vi "ExperimentProgramUI.vi"() -> ()   [LabVIEW 2011]
uses:
  Motors/MotorAxisEnum.ctl
  Motors/MotorPosType.ctl
  Typedefs/XYf.ctl
  Motors/MotorPosFlagsType.ctl
  Typedefs/MeasureConfigOutputMode.ctl
  Typedefs/CmdEnum_UserInterfaceCmd.ctl
  GlobalVariables.vi
panel:
  in  "Run sections util":bool
  in  "Run experiment":bool
  in  "Which motors should the script control?":T1={"Magnet Z"=TRUE, "Magnet rotation"=TRUE, "Camera"={"X"=FALSE, "Y"=FALSE}, "Piezo XY"={"X"=FALSE, "Y"=FALSE}, "Piezo Z"=FALSE}
  in  "Program.Motor Axis accuracy conditions":T2
  out "Simulated positions":T2[](array[typedef])
  in  "Axis to show in graph":T4[](array[typedef])=[enum."magrot", enum."magrot", enum."magpos"]
  out "Positions according to program":dbl[][](graph)
  in  "Tab Control 2":enum32{"Script", "MetaData", "Paths & Settings"}(tab)
  in  "Test run without experiment":bool
  in  "Script":string="% Initial position\n%move magpos 20; move magrot 0;\n%wait\n\n% Program\n%move magrot 1000 speed 100; wait;\n%move magrot 50 speed 10;\n%move magpos 10 speed 2;wait\n"
  in  "Simulate script":bool
  in  "Save script":bool
  in  "Load script":bool
  in  "Description":string
  in  "Project Name":string
  in  "Date":string
  in  "Researcher Name":string
  in  "Bead type":string
  in  "Protocol used":string
  in  "Notes":string
  in  "Write interval [frames]":i32
  in  "Experiment base path":path
  in  "Experiment name":string
  out "Traces will end up here:":path
  in  "Output mode":T5=enum."Track"
  in  "Image output path":string
  in  "Trace output path":string
  in  "Max frames in memory":i32
  out "Approx size in RAM memory:":string
  in  "stop":bool
  # "Axis names:\nmagrot:   Magnet rotation\nmagpos:   Magnet Z (vertical) position\npx, py, pz:   Piezo stage\ncamx, camy: Camera motorized stage\n\nScript events:\nSee bin/Modules/ScriptEventExample.vi"
  # "Instructions:\nmove <axis> <position>;\nMove axis to position at current speed\nmove <axis> <position> speed <speed>;\nMove axis to position at specified speed (units/s)\nidle <seconds>;\nDo nothing for specified time\nsection <optional name>;\nStore current framenumber in section file\nstop;\nStop experiment\nevent <text / parameters>;\nGenerate a script event (see left)"
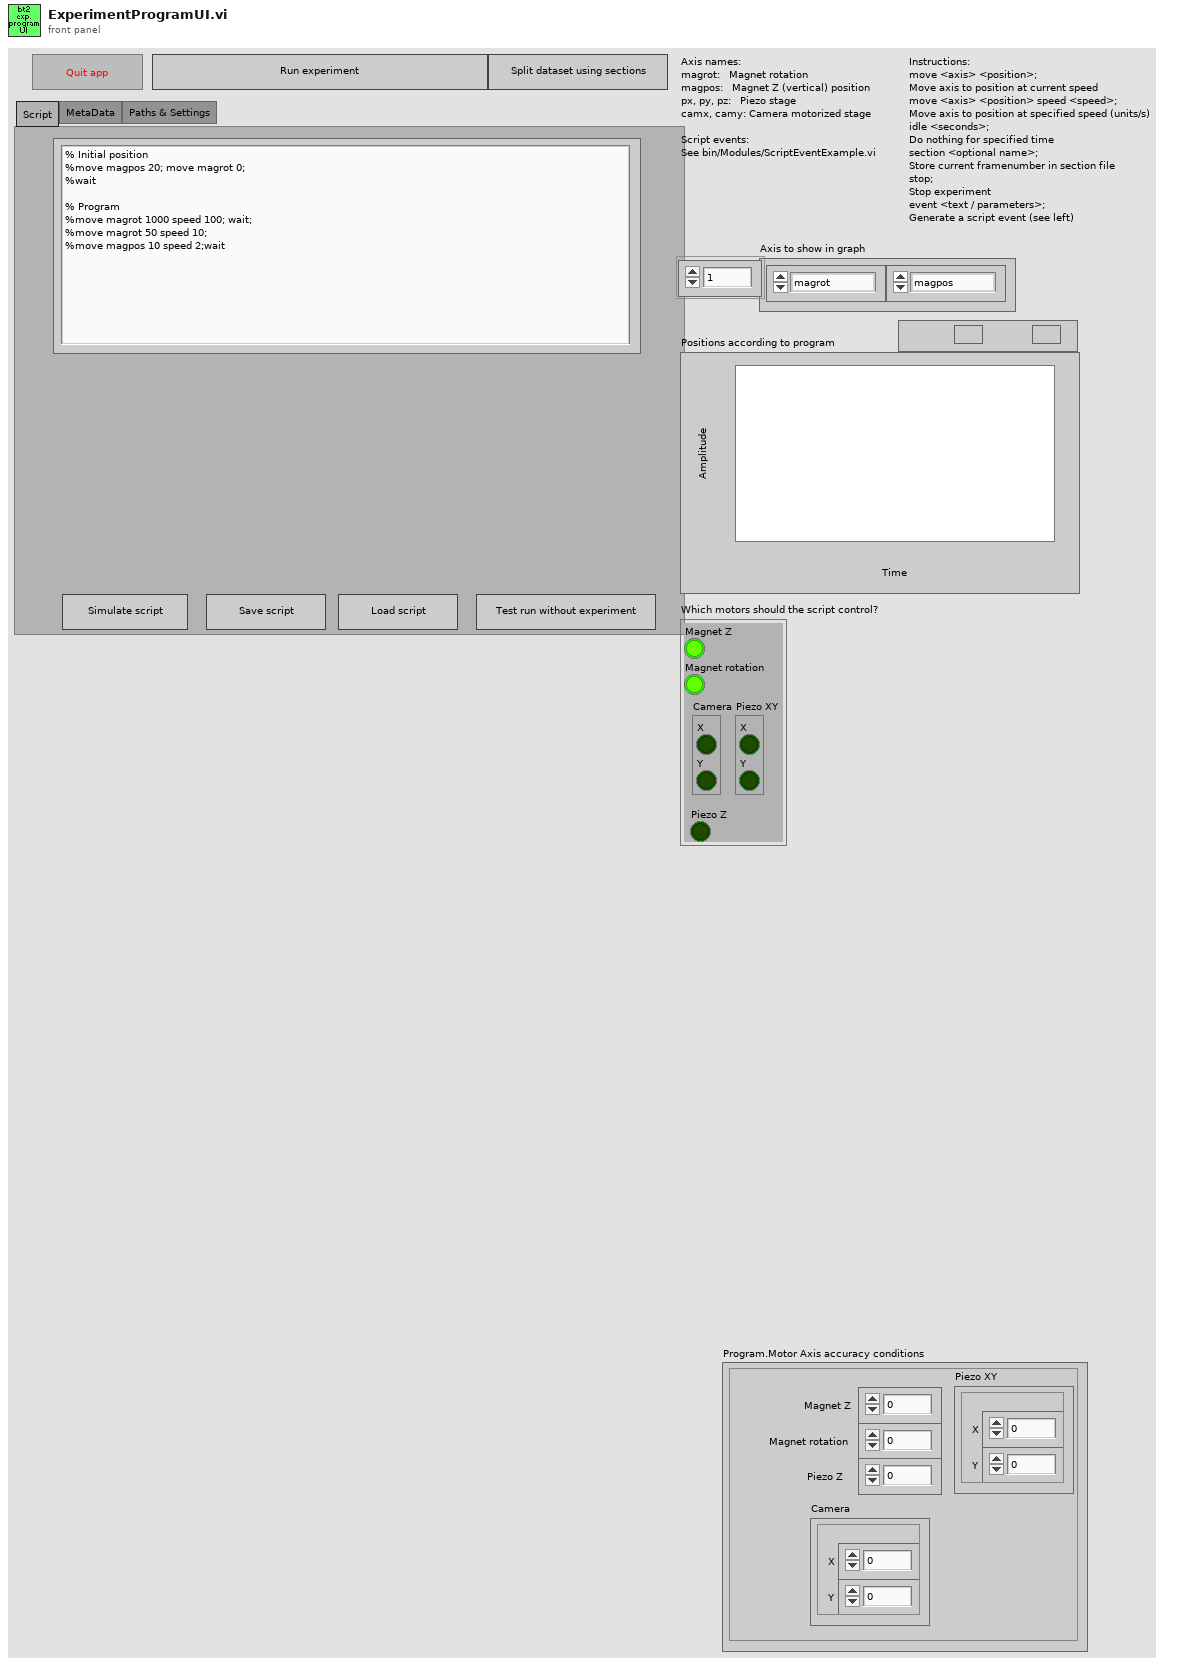
[diagram p1: front panel]
types:
  T1 = typedef "MotorPosFlagsType.ctl" = cluster{"Magnet Z":bool, "Magnet rotation":bool, "Camera":cluster{"X":bool, "Y":bool}, "Piezo XY":cluster{"X":bool, "Y":bool}, "Piezo Z":bool}
  T2 = typedef "MotorPosType.ctl" = cluster{"Magnet Z":dbl, "Magnet rotation":dbl, "Camera":T3, "Piezo XY":T3, "Piezo Z":dbl}
  T3 = typedef "XYf.ctl" = cluster{"X":sgl, "Y":sgl}
  T4 = typedef "MotorAxisEnum.ctl" = enum16{"no axis", "magrot", "magpos", "px", "py", "pz", "camx", "camy"}
  T5 = typedef "MeasureConfigOutputMode.ctl" = enum16{"None", "Track", "SaveImages"}
  T6 = cluster{"UpdateGraphEvent":refnum<user-event>, "MeasureConfigUpdated":refnum<user-event>}
  T7 = typedef "QueueListType.ctl" = cluster{"Motor In":refnum<queue>, "User Interface Image View":refnum<queue>, "User Interface Camera Control":refnum<queue>, "User Interface Event Notifier":refnum<notifier>, "Initialized?":bool, "Experiment Script Event Notifier":refnum<notifier>}
  T8 = typedef "CmdEnum_UserInterfaceCmd.ctl" = enum32{"Idle (Use for default)", "ResultTracesUpdated", "MeasureConfigUpdated", "MeasureEnd", "MeasureStart"}
  T9 = typedef "MeasureConfigType.ctl" = cluster{"Bead locations":cluster{"X":i32, "Y":i32}[], "ROI":i32, "Experiment base path":path, "Image output subdir":string, "Output mode":T5, "Traces output subdir":string, "QTrk Settings":T10, "Tracking Config":T11, "Experiment Name":string, "Program":T14, "ZLUT":sgl[][][], "Camera settings":T17, "Experiment Script":string, "Max frames in memory":i32, "Save traces as binary":bool, "Pixel Calibration Gain Image":string, "Pixel Calibration Offset Image":string, "Use pixel calibration images":bool, "Internal camera settings":string, "Trace write interval":i32, "ExperimentComment":string}
  T10 = typedef "QTrkSettings.ctl" = cluster{"Image width":i32, "Image height":i32, "Number of threads (CPU based)":i32, "CUDA Device":i32, "COM Background correction factor":sgl, "ZLUT MinRadius":sgl, "ZLUT Radial sample density":sgl, "ZLUT Angular sample density":sgl, "ZLUT ROI Coverage":sgl, "QI Iterations":i32, "QI MinRadius":sgl, "QI Radial sample density":sgl, "QI Angular sample density":sgl, "QI ROI Coverage":sgl, "QI Angular Step \nIteration Factor":sgl, "XCOR Profile Length":i32, "XCOR Profile Width":i32, "XCOR Iterations":i32, "Gaussian 2D Fit Iterations":i32, "Gaussian 2D Sigma (pixels)":sgl, "Downsample":i32}
  T11 = typedef "TrackingConfigType.ctl" = cluster{"Number of steps":i32, "ZLUT stepsize (um)":sgl, "Z correction factor":sgl, "Start piezo Z (um)":sgl, "Pixel size (nm)":sgl, "2D Localization Type":T12, "Z Command (None)":T13, "Z Piezo scale":bool, "ZLUT Building\nimages per frame":i32, "ZLUT Bias correction planes":i32}
  T12 = typedef "QTrkLocalizationType.ctl" = enum16{"Center-of-Mass", "1D Cross-Correlation", "Quadrant Interpolation", "Gaussian 2D MLE", "QI + ZLUTAlign", "ZLUTAlign", "QI + FourierLUT"}
  T13 = typedef "QTrkZCommandType.ctl" = enum16{"Nothing", "ComputeZ", "BuildRadialZLUT", "BuildImageZLUT", "RadialZLUT+ImageZLUT"}
  T14 = typedef "ExperimentProgramType.ctl" = cluster{"Commands":T15[], "Motor Axis accuracy conditions":T2, "Axis flags":T1}
  T15 = typedef "ExProgCommandType.ctl" = cluster{"cmd":T16, "axis":T4, "value/pos":dbl, "speed":dbl, "name":string}
  T16 = typedef "ExProgCommandEnumType.ctl" = enum16{"wait", "move", "event", "idle", "when", "section", "stop"}
  T17 = typedef "GenericCameraConfigType.ctl" = cluster{"Framerate (Hz)":i32, "Exposure time (us)":i32, "Image size":cluster{"Width":i32, "Height":i32}, "Number of buffers":i32}
  T18 = typedef "UserInterfaceEventType.ctl" = cluster{"Type":T8}
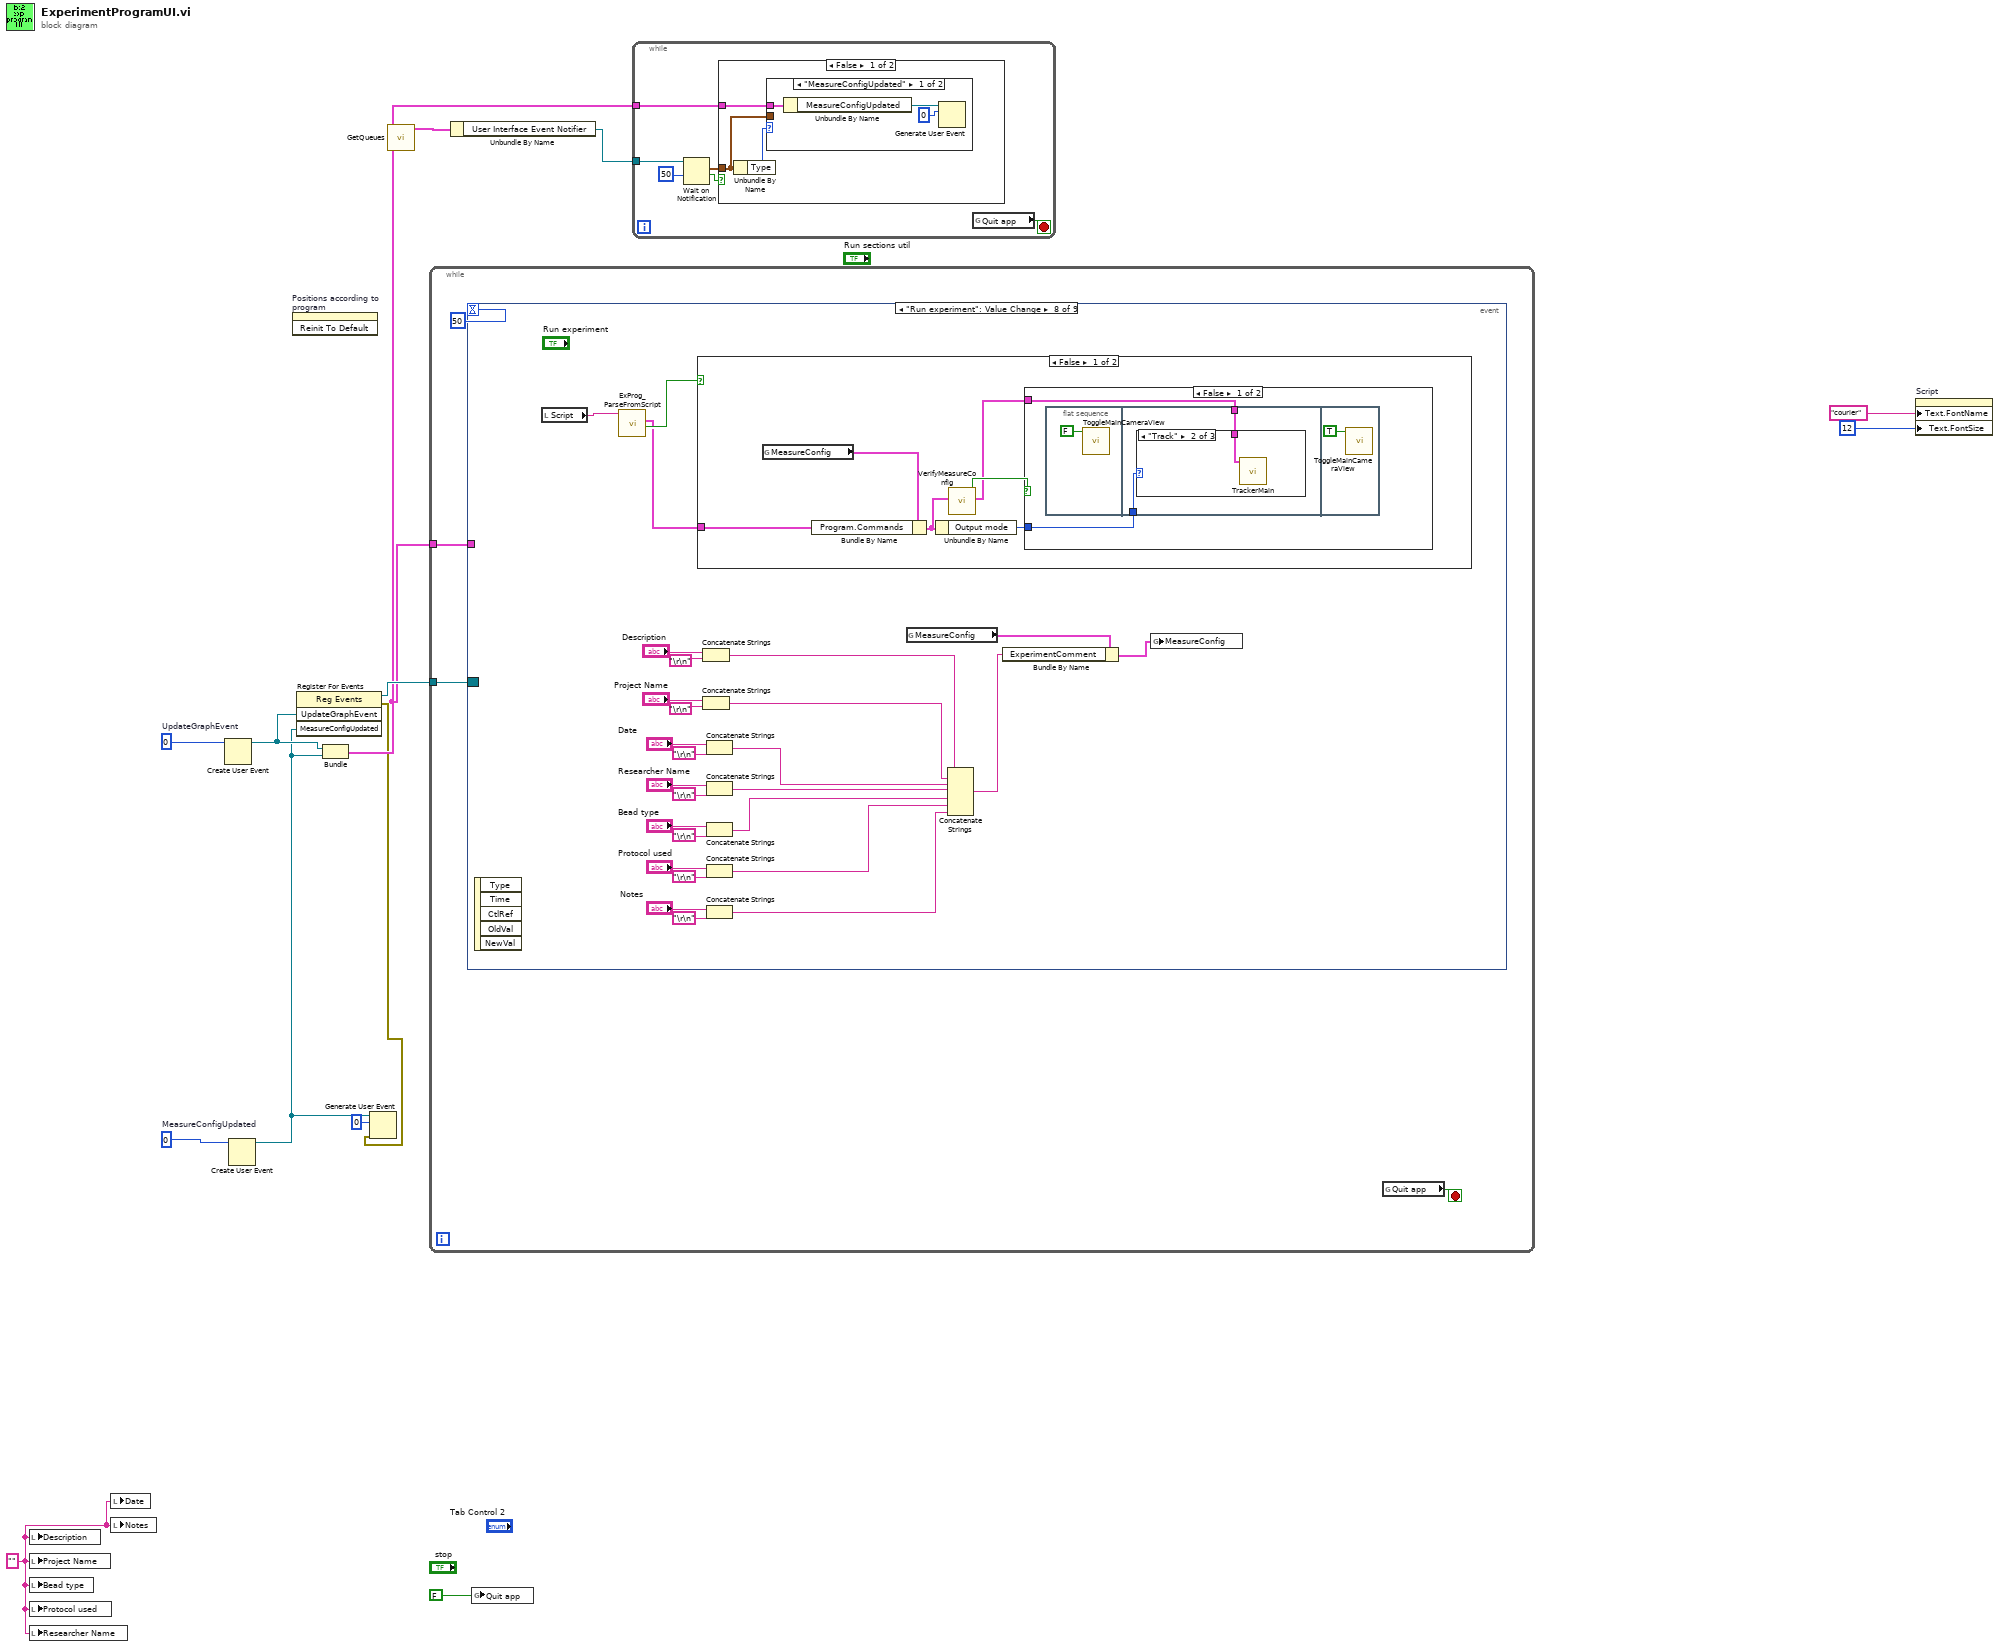
[diagram p0: block diagram]
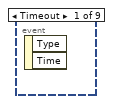
[diagram p4: hidden frame]
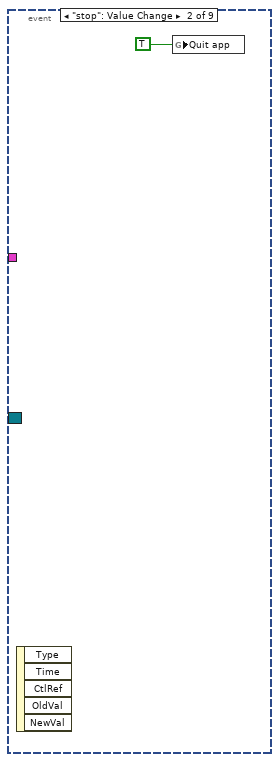
[diagram p5: hidden frame]
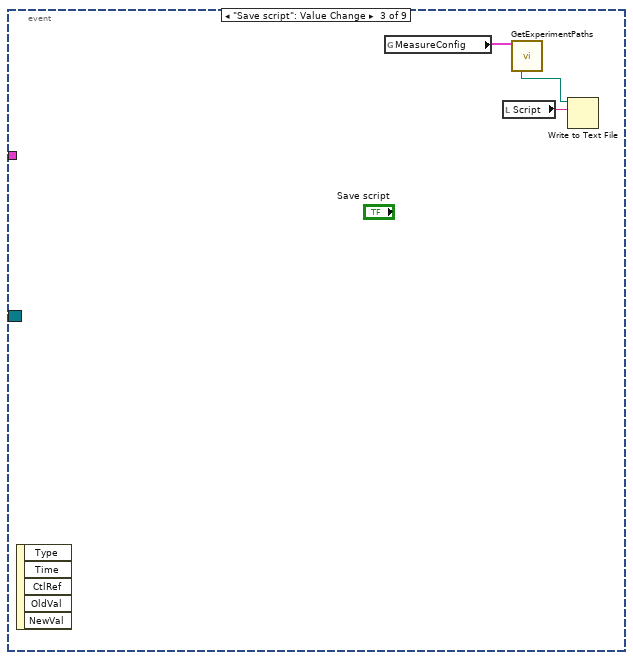
[diagram p6: hidden frame]
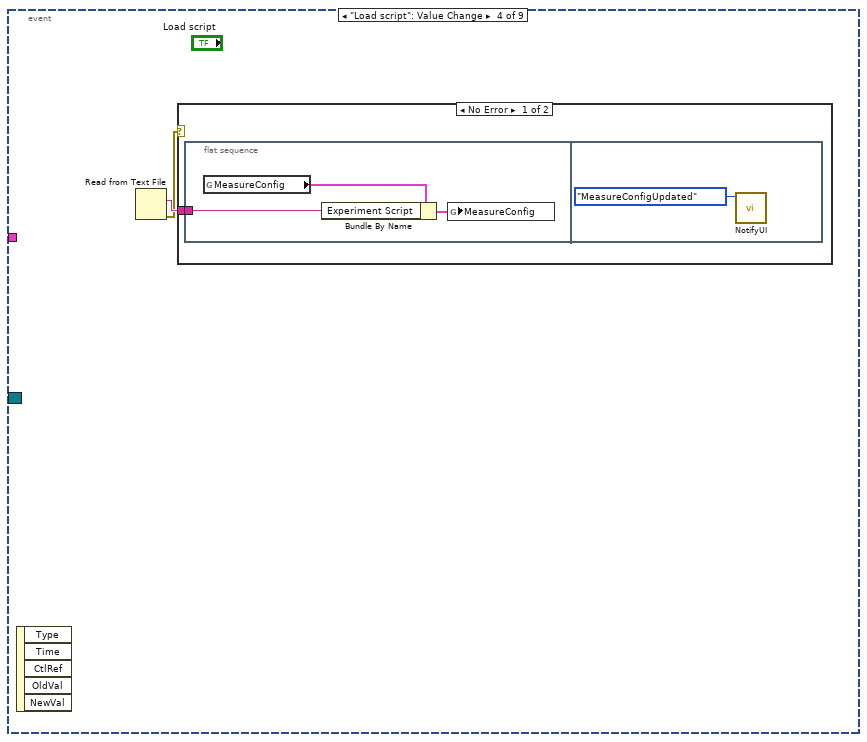
[diagram p7: hidden frame]
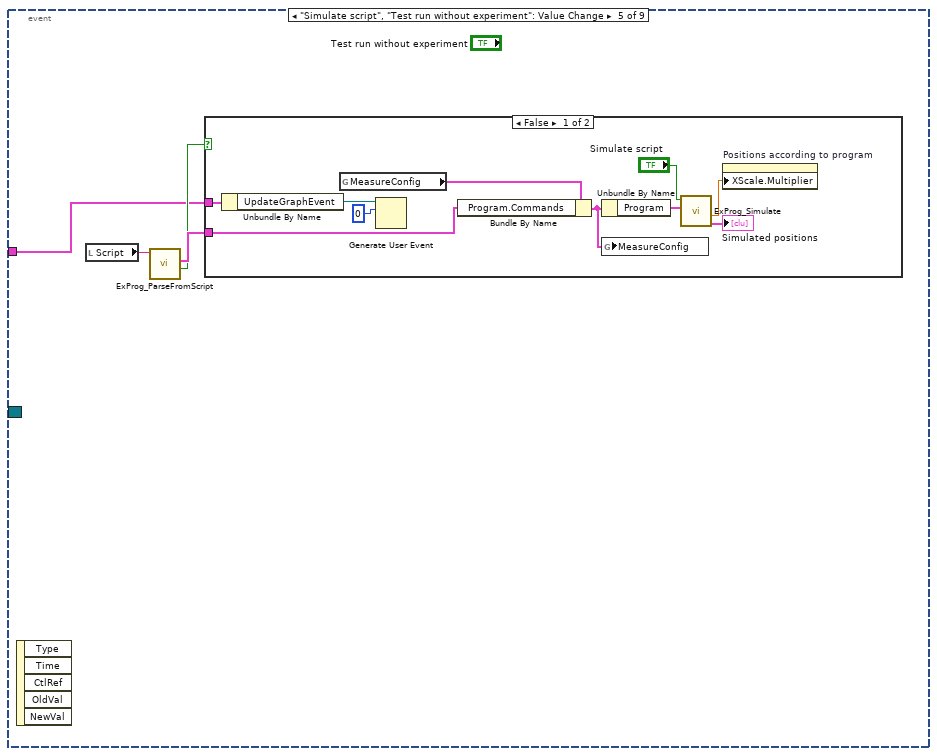
[diagram p9: hidden frame]
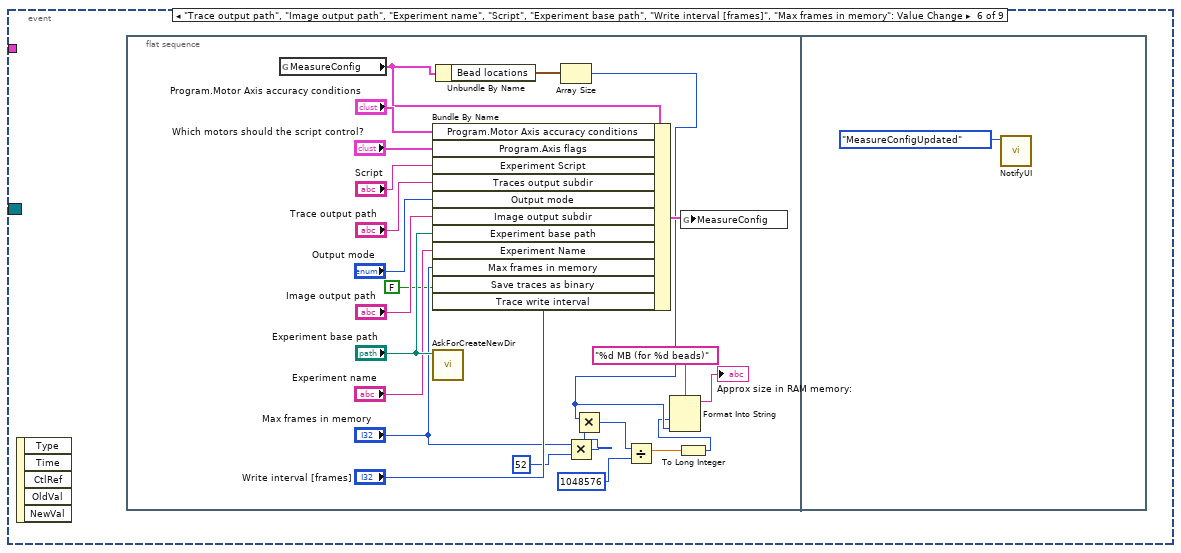
[diagram p11: hidden frame]
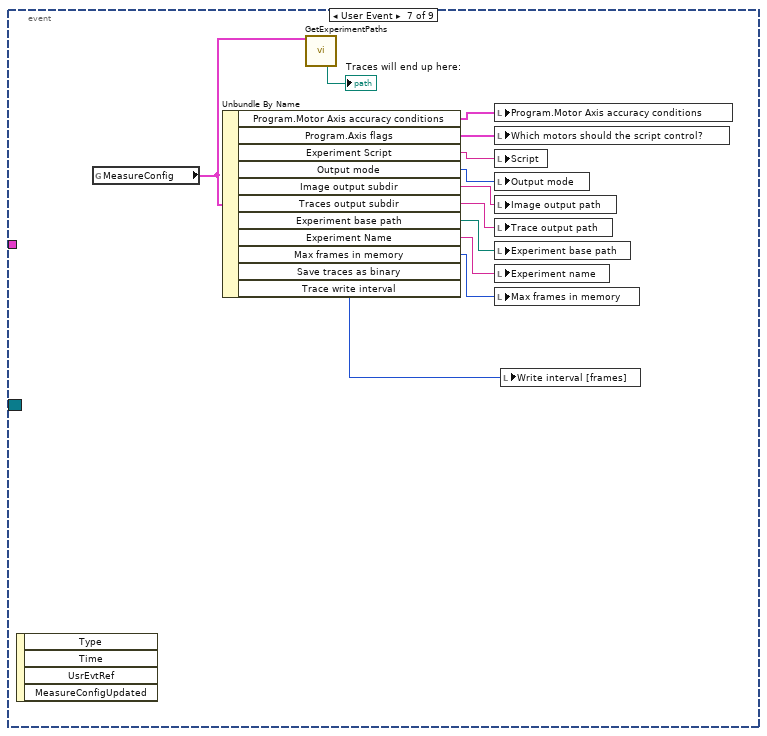
[diagram p12: hidden frame]
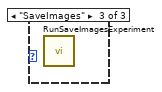
[diagram p14: hidden frame]
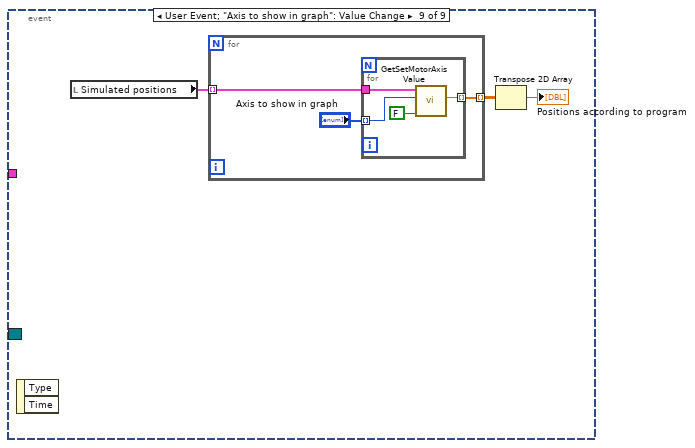
[diagram p17: hidden frame]
diagram:
  w1 = "" ("Description")
  w7 = 0  # MeasureConfigUpdated
  w9 = 0  # UpdateGraphEvent
  n1 = local write "Description"(w1) -> ()
  n2 = local write "Project Name"(w1) -> ()
  n3 = local write "Bead type"(w1) -> ()
  n4 = local write "Protocol used"(w1) -> ()
  n5 = local write "Researcher Name"(w1) -> ()
  n6 = local write "Date"(w1) -> ()
  n7 = local write "Notes"(w1) -> ()
  n8 = Create User Event(user event datatype=w9) -> (user event=w8:refnum<user-event>)  [unwired: 1 in, 1 out]
  n9 = Create User Event(user event datatype=w7) -> (user event=w5:refnum<user-event>)  [unwired: 1 in, 1 out]
  n10 = invoke on="Positions according to program" class="WFGraph (strict)" method="Reinit To Default"() -> ()  [unwired: 3 in, 3 out]
  n11 = register-events(w8, w5) -> (reference out=w10:refnum<event-registration>, error out=w3:errorcluster)  [unwired: 2 in]
  n12 = Bundle("UpdateGraphEvent"=w8, "MeasureConfigUpdated"=w5) -> (w6:T6)  [unwired: 1 in]
  n13 = Generate User Event(user event=w5, event data cluster=0 ("event data"), error in=w3) -> ()  [unwired: 2 out]
  n14 = call "GetQueues.vi"() -> ("Queue List"=w11:T7)  [unwired: 10 in, 1 out]
  n15 = while {
    tunnel: w10 -> [w16]
    tunnel: w6 -> [w15]
    stop <- w18 stop-if-true
    n16 = event shown="[7] \"Run experiment\": Value Change" {
      selector: w16 -> [_ _ _ _ _ _ _ _ _]
      dyn-events: _ -> [_ _ _ _ _ _ _ _ _]
      timeout: 50 -> [_ _ _ _ _ _ _ _ _]
      tunnel: w15 -> [_ _ _ _ w31 _ _ _ _]
      event Timeout {
        n17 = event-data() -> ()  [unwired: 1 in, 2 out]
      }
      event "stop": Value Change {
        n18 = event-data() -> ()  [unwired: 1 in, 5 out]
        n19 = global write "GlobalVariables.vi" "Quit app"(TRUE ("Quit app")) -> ()
      }
      event "Save script": Value Change {
        n20 = event-data() -> ()  [unwired: 1 in, 5 out]
        n21 = global read "GlobalVariables.vi" "MeasureConfig"() -> (w22:T9)
        n22 = local read "Script"() -> (w21:string)
        n23 = call "GetExperimentPaths.vi"("MeasureConfig"=w22) -> ("[base]\\[expname]_script.txt"=w20:path)  [unwired: 6 in, 8 out]
        n24 = Write to Text File(file (use dialog)=w20, text=w21) -> ()  [unwired: 2 in, 3 out]
      }
      event "Load script": Value Change {
        n25 = event-data() -> ()  [unwired: 1 in, 5 out]
        n26 = Read from Text File() -> (text=w24:string, error out=w23:errorcluster)  [unwired: 4 in, 2 out]
        n27 = case shown="No Error" w23 {
          tunnel: w24 -> [w25 _]
          frame No Error {
            n28 = flat-sequence {
              tunnel: w25 -> [w26]
              frame #0 {
                n29 = global read "GlobalVariables.vi" "MeasureConfig"() -> (w27:T9)
                n30 = Bundle By Name(cluster=w27, "Experiment Script"=w26) -> (w28:T9)
                n31 = global write "GlobalVariables.vi" "MeasureConfig"(w28) -> ()
              }
              frame #1 {
                n32 = call "NotifyUI.vi"("User Interface Commands"=CmdEnum_UserInterfaceCmd."MeasureConfigUpdated") -> ()  [unwired: 11 in]
              }
            }
          }
          frame Error {
          }
        }
      }
      event "Simulate script", "Test run without experiment": Value Change {
        n33 = event-data() -> ()  [unwired: 1 in, 5 out]
        n34 = local read "Script"() -> (w30:string)
        n35 = call "ExProg_ParseFromScript.vi"("text"=w30) -> ("error?"=w32:bool, "program"=w33:T15[])  [unwired: 9 in]
        n36 = case shown="False" w32 {
          tunnel: w33 -> [w42 _]
          tunnel: w31 -> [w38 _]
          frame False {
            n37 = Unbundle By Name(w38) -> ("UpdateGraphEvent"=w37:refnum<user-event>)
            n38 = global read "GlobalVariables.vi" "MeasureConfig"() -> (w43:T9)
            n39 = Generate User Event(user event=w37, event data cluster=0 ("event data")) -> ()  [unwired: 1 in, 2 out]
            n40 = Bundle By Name(cluster=w43, "Program.Commands"=w42) -> (w41:T9)
            n41 = Unbundle By Name(w41) -> ("Program"=w40:T14)
            n42 = global write "GlobalVariables.vi" "MeasureConfig"(w41) -> ()
            n43 = call "ExProg_Simulate.vi"("Program"=w40, "Simulation?"="Simulate script") -> ("Wanted position list"=→"Simulated positions":T2[], "Used timestep (s)"=w39:sgl)  [unwired: 8 in]
            n44 = property on="Positions according to program" class="WFGraph (strict)"("XScale.Multiplier"=w39) -> ()  [unwired: 2 in, 2 out]
          }
          frame True {
          }
        }
      }
      event "Trace output path", "Image output path", "Experiment name", "Script", "Experiment base path", "Write interval [frames]", "Max frames in memory": Value Change {
        n45 = event-data() -> ()  [unwired: 1 in, 5 out]
        n46 = flat-sequence {
          frame #0 {
            n47 = global read "GlobalVariables.vi" "MeasureConfig"() -> (w52:T9)
            n48 = Bundle By Name(cluster=w52, "Program.Motor Axis accuracy conditions"="Program.Motor Axis accuracy conditions", "Program.Axis flags"="Which motors should the script control?", "Experiment Script"="Script", "Traces output subdir"="Trace output path", "Output mode"="Output mode", "Image output subdir"="Image output path", "Experiment base path"="Experiment base path", "Experiment Name"="Experiment name", "Max frames in memory"="Max frames in memory", "Save traces as binary"=FALSE, "Trace write interval"="Write interval [frames]") -> (w66:T9)
            n49 = call "AskForCreateNewDir.vi"("Experiment base path"="Experiment base path") -> ()  [unwired: 11 in]
            n50 = Unbundle By Name(w52) -> ("Bead locations"=w51:cluster{"X":i32, "Y":i32}[])
            n51 = Array Size(array=w51) -> (size(s)=w47:i32)
            n52 = Multiply(x="Max frames in memory", y=52) -> (x*y=w50:i32)
            n53 = Multiply(x=w47, y=w50) -> (x*y=w49:i32)
            n54 = Divide(x=w49, y=1048576) -> (x/y=w54:dbl)
            n55 = To Long Integer(number=w54) -> (32bit integer=w46:i32)
            n56 = Format Into String(format string="%d MB (for %d beads)", w46, w47) -> (resulting string=→"Approx size in RAM memory:":string)  [unwired: 2 in, 1 out]
            n57 = global write "GlobalVariables.vi" "MeasureConfig"(w66) -> ()
          }
          frame #1 {
            n58 = call "NotifyUI.vi"("User Interface Commands"=CmdEnum_UserInterfaceCmd."MeasureConfigUpdated") -> ()  [unwired: 11 in]
          }
        }
      }
      event User Event {
        n59 = event-data() -> ()  [unwired: 1 in, 4 out]
        n60 = global read "GlobalVariables.vi" "MeasureConfig"() -> (w73:T9)
        n61 = Unbundle By Name(w73) -> ("Program.Motor Axis accuracy conditions"=w79:T2, "Program.Axis flags"=w78:T1, "Experiment Script"=w77:string, "Output mode"=w76:T5, "Image output subdir"=w75:string, "Traces output subdir"=w74:string, "Experiment base path"=w71:path, "Experiment Name"=w70:string, "Max frames in memory"=w69:i32, "Trace write interval"=w68:i32)  [unwired: 1 out]
        n62 = call "GetExperimentPaths.vi"("MeasureConfig"=w73) -> ("[base]\\traces\\[expname].txt/bin"=→"Traces will end up here:":path)  [unwired: 6 in, 8 out]
        n63 = local write "Program.Motor Axis accuracy conditions"(w79) -> ()
        n64 = local write "Which motors should the script control?"(w78) -> ()
        n65 = local write "Script"(w77) -> ()
        n66 = local write "Output mode"(w76) -> ()
        n67 = local write "Image output path"(w75) -> ()
        n68 = local write "Trace output path"(w74) -> ()
        n69 = local write "Experiment base path"(w71) -> ()
        n70 = local write "Experiment name"(w70) -> ()
        n71 = local write "Max frames in memory"(w69) -> ()
        n72 = local write "Write interval [frames]"(w68) -> ()
      }
      event "Run experiment": Value Change {
        n73 = event-data() -> ()  [unwired: 1 in, 5 out]
        n74 = local read "Script"() -> (w106:string)
        n75 = call "ExProg_ParseFromScript.vi"("text"=w106) -> ("error?"=w105:bool, "program"=w104:T15[])  [unwired: 9 in]
        n76 = case shown="False" w105 {
          tunnel: w104 -> [w110 _]
          frame False {
            n77 = global read "GlobalVariables.vi" "MeasureConfig"() -> (w111:T9)
            n78 = Bundle By Name(cluster=w111, "Program.Commands"=w110) -> (w108:T9)
            n79 = Unbundle By Name(w108) -> ("Output mode"=w112:T5)
            n80 = call "VerifyMeasureConfig.vi"("MeasureConfig"=w108) -> ("MeasureConfig 2"=w107:T9, "Cancel button pressed?"=w109:bool)  [unwired: 9 in]
            n81 = case shown="False" w109 {
              tunnel: w112 -> [w114 _]
              tunnel: w107 -> [w113 _]
              frame False {
                n82 = flat-sequence {
                  tunnel: w114 -> [w117]
                  tunnel: w113 -> [w116]
                  frame #0 {
                    n83 = call "ToggleMainCameraView.vi"("Enable? (T)"=FALSE) -> ()  [unwired: 11 in]
                  }
                  frame #1 {
                    n84 = case shown="\"Track\"" w117 {
                      tunnel: w116 -> [_ w118 _]
                      frame "None", Default {
                      }
                      frame "Track" {
                        n85 = call "TrackerMain.vi"("MeasureConfig"=w118) -> ()  [unwired: 10 in, 1 out]
                      }
                      frame "SaveImages" {
                        n86 = call "RunSaveImagesExperiment.vi"() -> ()  [unwired: 12 in]
                      }
                    }
                  }
                  frame #2 {
                    n87 = call "ToggleMainCameraView.vi"("Enable? (T)"=TRUE) -> ()  [unwired: 11 in]
                  }
                }
              }
              frame True {
              }
            }
          }
          frame True {
          }
        }
        n88 = Concatenate Strings("Description", "\r\n") -> (w99:string)
        n89 = Concatenate Strings("Project Name", "\r\n") -> (w92:string)
        n90 = Concatenate Strings("Date", "\r\n") -> (w91:string)
        n91 = Concatenate Strings("Researcher Name", "\r\n") -> (w90:string)
        n92 = Concatenate Strings("Bead type", "\r\n") -> (w89:string)
        n93 = Concatenate Strings("Protocol used", "\r\n") -> (w88:string)
        n94 = Concatenate Strings("Notes", "\r\n") -> (w87:string)
        n95 = global read "GlobalVariables.vi" "MeasureConfig"() -> (w103:T9)
        n96 = Concatenate Strings(w99, w92, w91, w90, w89, w88, w87) -> (w101:string)
        n97 = Bundle By Name(cluster=w103, "ExperimentComment"=w101) -> (w102:T9)
        n98 = global write "GlobalVariables.vi" "MeasureConfig"(w102) -> ()
      }
      event User Event; "Axis to show in graph": Value Change {
        n99 = event-data() -> ()  [unwired: 1 in, 2 out]
        n100 = local read "Simulated positions"() -> (w122:T2[])
        n101 = for {
          tunnel: w122 -> [w124] mode=indexing
          tunnel: [w123] -> w121 mode=indexing
          n102 = for {
            tunnel: "Axis to show in graph" -> [w128] mode=indexing
            tunnel: w124 -> [w129]
            tunnel: [w126] -> w123 mode=indexing
            n103 = call "GetSetMotorAxisValue.vi"("set? (T)"=FALSE, "axis"=w128, "Motorpos in"=w129) -> ("pos (out)"=w126:dbl)  [unwired: 7 in, 1 out]
          }
        }
        n104 = Transpose 2D Array(2D array=w121) -> (transposed array=→"Positions according to program":dbl[][])
      }
    }
    n105 = global read "GlobalVariables.vi" "Quit app"() -> (w18:bool)
  }
  n106 = Unbundle By Name(w11) -> ("User Interface Event Notifier"=w2:refnum<notifier>)
  n107 = global write "GlobalVariables.vi" "Quit app"(FALSE ("Quit app")) -> ()
  n108 = while {
    tunnel: w6 -> [w134]
    tunnel: w2 -> [w133]
    stop <- w135 stop-if-true
    n109 = Wait on Notification(notifier=w133, timeout in ms (-1)=50) -> (notification=w132:T18, timed out?=w130:bool)  [unwired: 2 in, 2 out]
    n110 = case shown="False" w130 {
      tunnel: w134 -> [w138 _]
      tunnel: w132 -> [w137 _]
      frame False {
        n111 = Unbundle By Name(w137) -> ("Type"=w136:T8)
        n112 = case shown="\"MeasureConfigUpdated\"" w136 {
          tunnel: w137 -> [_ _]
          tunnel: w138 -> [w141 _]
          frame "MeasureConfigUpdated" {
            n113 = Unbundle By Name(w141) -> ("MeasureConfigUpdated"=w140:refnum<user-event>)
            n114 = Generate User Event(user event=w140, event data cluster=0 ("event data")) -> ()  [unwired: 1 in, 2 out]
          }
          frame "Idle (Use for default)", Default {
          }
        }
      }
      frame True {
      }
    }
    n115 = global read "GlobalVariables.vi" "Quit app"() -> (w135:bool)
  }
  n116 = property on="Script" class="Str"("Text.FontName"="courier" ("Text.Font:Name"), "Text.FontSize"=u32 12 ("Text.Font:Size")) -> ()  [unwired: 2 in, 2 out]
